vi "server.Check Server Status.vi"(8 "error in (no error)":errorcluster, 11 "Request in":refnum<class "JSONRPC Server.lvclass">) -> (0 "error out":errorcluster, 2 "Server Running?":bool, 3 "Request out":refnum<class "JSONRPC Server.lvclass">)   [LabVIEW 2016, in "JSONRPC Server.lvclass"]
doc: "Checks to see if the Server Reference is still valid."
uses:
  JSONRPC Server.lvclass
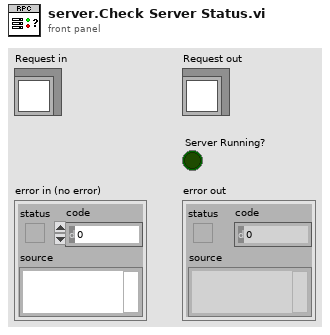
[diagram p1: front panel]
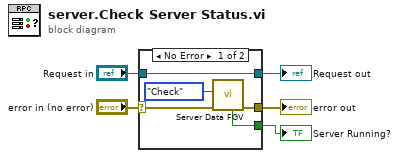
[diagram p0: block diagram]
diagram:
  n1 = case shown="No Error" "error in (no error)" {
    selector: "error in (no error)" -> [w8 w12]
    tunnel: [w7 w12] -> w4
    tunnel: [w10 w11] -> w2
    tunnel: "Request in" -> [w10 w11]
    tunnel: [w9 _] -> w1
    frame No Error {
      n2 = call "Server Data FGV.vi"("error in (no error)"=w8, "Action"=enum16{"Initialize", "Check", "Close"}."Check") -> ("error out"=w7:errorcluster, "Server Running"=w9:bool)  [unwired: 6 in, 2 out]
    }
    frame Error {
    }
  }
  "error out" <- w4
  "Request out" <- w2
  "Server Running?" <- w1
